vi "DockSubPanel.vi"(8 "ErrorIn":errorcluster, 9 "ObjectLabel":string, 10 "PanelLabel":string, 11 "ReferenceIn":refnum<class "MasterGUI.lvclass">) -> (0 "ErrorOut":errorcluster, 3 "ReferenceIn":refnum<class "MasterGUI.lvclass">)   [LabVIEW 2021, in "MasterGUI.lvclass"]
uses:
  MasterGUI.lvclass
  Interface_UserInterface_IFrontPanel/IFrontPanel/IFrontPanel.lvclass
  16f1a312-48ec-4227-8a7b-c00f47d308a5.vi
  <vilib>/TriekselSoft/TracerLibrary/TracerLibrary/Tracer/protected/SendMessage.vi
  <vilib>/TriekselSoft/TracerLibrary/TracerLibrary/Tracer/protected/Timestamp.vi
  16f1a312-48ec-4227-8a7b-c00f47d308a5.vi/f75db090-0877-4668-94fb-75c2140b1617.vi
  <vilib>/TriekselSoft/TracerLibrary/TracerLibrary/Tracer/Tracer_Level-Info.vi
  <vilib>/JDP Science/JSONtext/Variant to JSON Text.vi
  <vilib>/TriekselSoft/TracerLibrary/TracerLibrary/Tracer/protected/Tracer_ClassAttributes.vi
  <vilib>/JDP Science/JSONtext/LVClass Serializer/JSONtext LVClass Serializer.lvclass
  Library_UserInterface_FrontPanelControl/FrontPanelControl/FrontPanelControl.lvclass
  MasterGUI.lvclass/MasterGUI.ctl
  Application/Application.lvclass
  C:/Localdata/Projects/TriekselSoft/TriekselsoftApplicationFramework/Source/.Externals/Interface_UserInterface_IFrontPanel/IFrontPanel/IFrontPanel.lvclass
  C:/Localdata/Projects/TriekselSoft/TriekselsoftApplicationFramework/Source/IInterface/IInterface.lvclass
panel:
  # "s"
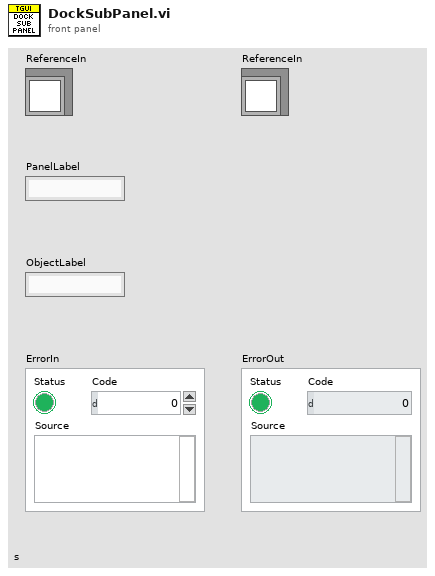
[diagram p1: front panel]
types:
  T1 = typedef "MasterGUI.lvclass/ObjectAttributes.ctl" = cluster{"Interfaces":cluster{"Dummy":refnum<class>}, "Locals":cluster{"MainGUIActive":refnum<queue>, "MainPanel":refnum<vi>, "LayoutPanel":cluster{"PanelVIRef":refnum<vi>, "Labels":string[], "SubPanels":refnum<vi>[]}, "MenuTree":T2[], "Menu":refnum<k9>}, "Persistent":cluster{"StaticDocking":cluster{"ObjectLabel":string, "SubPanelLabel":string}[], "WindowsTitle":string, "AdditionalMenuItems":T2[], "TraceObjectName":string}}
  T2 = typedef "MasterGUI.lvclass/MenuItem.ctl" = cluster{"Parent":string, "Items":string[], "ShortCuts":cluster{"IncludeShiftKey":bool, "IncludeCtrlKey":bool, "ShortcutKey":string}[]}
  T3 = cluster{"PanelLabel":string, "ObjectLabel":string}
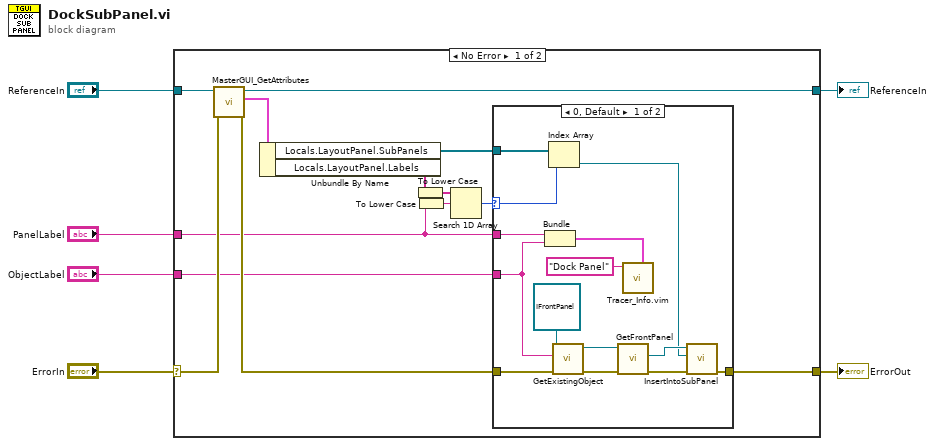
[diagram p0: block diagram]
diagram:
  n1 = case shown="No Error" "ErrorIn" {
    selector: "ErrorIn" -> [w19 w36]
    tunnel: [w17 w36] -> w5
    tunnel: [w14 w35] -> w3
    tunnel: "ReferenceIn" -> [w15 w35]
    tunnel: "PanelLabel" -> [w7 _]
    tunnel: "ObjectLabel" -> [w9 _]
    frame No Error {
      n2 = call "MasterGUI_GetAttributes.vi"("error in (no error)"=w19, "reference in"=w15) -> ("error out"=w18:errorcluster, "Data"=w16:T1, "reference out"=w14:refnum<class "MasterGUI.lvclass">)  [unwired: 6 in, 1 out]
      n3 = Unbundle By Name(w16) -> ("Locals.LayoutPanel.SubPanels"=w8:refnum<vi>[], "Locals.LayoutPanel.Labels"=w13:string[])
      n4 = To Lower Case(string=w13) -> (all lower case string=w12:string[])
      n5 = To Lower Case(string=w7) -> (all lower case string=w11:string)
      n6 = Search 1D Array(1D array=w12, element=w11) -> (index of element=w10:i32)  [unwired: 1 in]
      n7 = case shown="0, Default" w10 {
        selector: w10 -> [w26 _]
        tunnel: [w30 w34] -> w17
        tunnel: w18 -> [w33 w34]
        tunnel: w9 -> [w24 _]
        tunnel: w8 -> [w27 _]
        tunnel: w7 -> [w25 _]
        frame 0, Default {
          n8 = Bundle("PanelLabel"=w25, "ObjectLabel"=w24) -> (w23:T3)  [unwired: 1 in]
          n9 = Index Array(array=w27, index=w26) -> (element=w20:refnum<vi>)
          n10 = call "GetExistingObject.vi"("ErrorIn"=w33, "ObjectName"=w24, "Type"=refnum<class "IFrontPanel.lvclass"> refnum ("IFrontPanel")) -> ("ErrorOut"=w32:errorcluster, "ObjectOut"=w28:refnum<class "IFrontPanel.lvclass">)  [unwired: 7 in]
          n11 = call-dynamic "GetFrontPanel.vi"("ErrorIn"=w32, "ObjectIn"=w28) -> ("ErrorOut"=w31:errorcluster, "FrontPanelControl"=w21:refnum<class "FrontPanelControl.lvclass">)  [unwired: 7 in, 1 out]
          n12 = call "Tracer_Info.vim"("Data"=w23, "InfoText"="Dock Panel") -> ()  [unwired: 9 in, 1 out]
          n13 = call-dynamic "InsertIntoSubPanel.vi"("Error In"=w31, "SubPanel in"=w20, "object in"=w21) -> ("Error Out"=w30:errorcluster)  [unwired: 7 in, 1 out]
        }
        frame -1 {
        }
      }
    }
    frame Error {
    }
  }
  "ErrorOut" <- w5
  "ReferenceIn" <- w3
